vi "Get Random Name.vi"() -> (0 "random Name":string)   [LabVIEW 2021, in "Architecture.lvlib" / "Message.lvclass"]
doc: "Obtain a random name to be used as queue names or event names"
uses:
  Message.lvclass
  Message.lvclass/Message.ctl
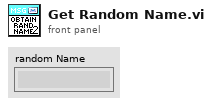
[diagram p1: front panel]
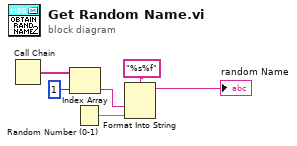
[diagram p0: block diagram]
diagram:
  n1 = Call Chain() -> (call chain=w2:string[])
  n2 = Index Array(array=w2, index=1) -> (element=w4:string)
  n3 = Random Number (0-1)() -> (number: 0 to 1=w6:dbl)
  n4 = Format Into String(format string="%s%f", w4, w6) -> (resulting string=→"random Name":string)  [unwired: 2 in, 1 out]
